vi "Begin.vi"(11 "Image Size":T1=enum."160x120") -> (0 "error out":errorcluster)   [LabVIEW 2012]
doc: "Called before other user functions, this VI is expected to open initial I/O refnums, load in file data, and do all program initialization. Notice that the <B>error out</B> terminal is simply used for data flow. Wiring it to other structures or subVIs ensures that this VI runs first."
uses:
  <vilib>/Rock Robotics/WPI/Camera/WPI_CameraImageSize.ctl
  <vilib>/Rock Robotics/SystemInterfaces/DIO/FPGA_DIOPWMChannel.ctl
  <vilib>/Rock Robotics/WPI/Joystick/WPI_JoystickDeviceEnum.ctl
  <vilib>/Rock Robotics/WPI/Camera/WPI_CameraWhite Balance Values.ctl
  <vilib>/Rock Robotics/WPI/Camera/WPI_CameraExposure Values.ctl
  <vilib>/Rock Robotics/WPI/Camera/WPI_CameraFrameRate.ctl
  <vilib>/Rock Robotics/SystemInterfaces/DIO/FPGA_DIOChannel.ctl
  <vilib>/Rock Robotics/SystemInterfaces/Typedef/FPGA_TypedefDigitalModule.ctl
  <vilib>/Rock Robotics/WPI/Encoder/WPI_EncoderType.ctl
  <vilib>/Rock Robotics/SystemInterfaces/DIO/FPGA_DIORelayChannel.ctl
  <vilib>/Rock Robotics/SystemInterfaces/Typedef/FPGA_TypedefAnalogModuleForGyro.ctl
  <vilib>/Rock Robotics/SystemInterfaces/AI/FPGA_AIGyroChannel.ctl
  <vilib>/Rock Robotics/WPI/Relay/WPI_RelayDirection.ctl
  <vilib>/Rock Robotics/WPI/MotorControl/WPI_MotorControlOpen Victor.vi
  <vilib>/Rock Robotics/WPI/RobotDrive/WPI_RobotDriveOpen4MotorWithJaguar.vi
  Robot Global Data.vi
  <vilib>/Rock Robotics/WPI/Counter/WPI_CounterOpen UpDown Mode.vi
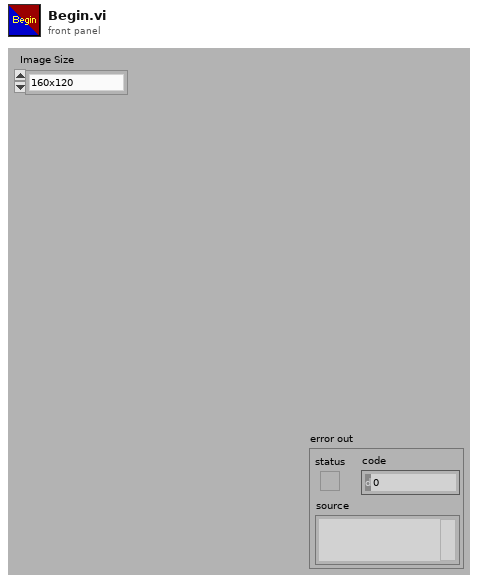
[diagram p1: front panel]
types:
  T1 = typedef "WPI_CameraImageSize.ctl" = enum16{"640x480", "320x240", "160x120"}
  T2 = typedef "FPGA_TypedefDigitalModule.ctl" = enum16{"Digital Module 1", "Digital Module 2"}
  T3 = typedef "FPGA_DIOChannel.ctl" = enum8{"DIO 1", "DIO 2", "DIO 3", "DIO 4", "DIO 5", "DIO 6", "DIO 7", "DIO 8", "DIO 9", "DIO 10", "DIO 11", "DIO 12", "DIO 13", "DIO 14", "Invalid"}
  T4 = typedef "WPI_RelayDirection.ctl" = enum16{"Both directions", "Forward only", "Reverse only"}
  T5 = typedef "FPGA_AIGyroChannel.ctl" = enum8{"AI 1", "AI 2", "Invalid"}
  T6 = typedef "FPGA_TypedefAnalogModuleForGyro.ctl" = enum16{"Analog Module 1"}
  T7 = typedef "FPGA_DIORelayChannel.ctl" = enum8{"Relay 1", "Relay 2", "Relay 3", "Relay 4", "Relay 5", "Relay 6", "Relay 7", "Relay 8", "Invalid"}
  T8 = typedef "WPI_EncoderType.ctl" = enum16{"1x", "2x", "4x"}
  T9 = typedef "FPGA_DIOPWMChannel.ctl" = enum8{"PWM 1", "PWM 2", "PWM 3", "PWM 4", "PWM 5", "PWM 6", "PWM 7", "PWM 8", "PWM 9", "PWM 10", "Invalid"}
  T10 = typedef "WPI_JoystickDeviceEnum.ctl" = enum16{"USB 1", "USB 2", "USB 3", "USB 4", "Kinect 1", "Kinect 2"}
  T11 = typedef "WPI_CameraFrameRate.ctl" = u32
  T12 = typedef "WPI_CameraExposure Values.ctl" = enum16{"Auto", "Flicker-free 50 Hz", "Flicker-free 60 Hz", "Hold current"}
  T13 = typedef "WPI_CameraWhite Balance Values.ctl" = enum16{"Auto", "Fixed indoor", "Fixed outdoor 1", "Fixed outdoor 2", "Fixed fluorescent 1", "Fixed fluorescent 2", "Hold current"}
  T14 = typedef "WPI_CameraDevRef.ctl" = cluster{"Camera Address":string, "CameraStatus":errorcluster, "Acquire Image Notifier":refnum<notifier>}
  T15 = typedef "WPI_DigitalInputDevRef.ctl" = cluster{"DevStatus":errorcluster, "DIO Channel":T3, "Digital Module":T2}
  T16 = typedef "WPI_RobotDriveDevRef.ctl" = cluster{"DevStatus":errorcluster, "Motors[]":T17[], "Square Inputs":bool, "Max Output":dbl, "Isochronous":bool}
  T17 = typedef "WPI_MotorControlDeviceRef.ctl" = cluster{"DeviceStatus":errorcluster, "Type":enum16{"PWM", "CAN"}, "PWM":cluster{"Digital Module":T2, "PWM Channel":T9, "DeadBand":T18}, "CAN":cluster{"Device Number":u8, "Control Mode":T19, "Semaphore":T20, "Max Vout":dbl}, "Invert":bool, "TransformRef":T21, "InvTransformRef":T21}
  T18 = typedef "WPI_PWMDeadband.ctl" = cluster{"Name":string, "maxPositivePwm":i32, "minPositivePwm":i32, "centerPwm":i32, "maxNegativePwm":i32, "minNegativePwm":i32, "angularRange":u16}
  T19 = typedef "WPI_CANJaguar_ControlMode.ctl" = enum8{"Percent VBus", "Current", "Speed", "Position", "Voltage"}
  T20 = typedef "Semaphore RefNum" = refnum<k1>
  T21 = typedef "WPI_PWMTransform_ConPane.ctl" = refnum<vi>
  T22 = typedef "FPGA_CounterEncoderSourceConvertionLVSourceType.ctl" = cluster{"DevStatus":errorcluster, "AnalogTriggerMode?":bool, "DigitalMode":cluster{"Digital Module":T2, "DIO Channel":T23}, "AnalogTriggerMode":cluster{"AnalogTriggerIndex":T24, "OutputType":T25}}
  T23 = typedef "FPGA_DIODigitalSourceChannel.ctl" = enum8{"DIO 1", "DIO 2", "DIO 3", "DIO 4", "DIO 5", "DIO 6", "DIO 7", "DIO 8", "DIO 9", "DIO 10", "DIO 11", "DIO 12", "DIO 13", "DIO 14", "Disabled"}
  T24 = typedef "FPGA_AnalogTriggerIndex.ctl" = enum8{"Trig 0", "Trig 1", "Trig 2", "Trig 3", "Trig 4", "Trig 5", "Trig 6", "Trig 7", "Invalid"}
  T25 = typedef "FPGA_AnalogTriggerOutType.ctl" = enum16{"InWindow", "TriggerState", "Rising", "Falling"}
  T26 = typedef "WPI_GyroDevRef.ctl" = cluster{"DevStatus":errorcluster, "Analog Module":T27, "Analog Channel":T28, "Offset":dbl, "Gain (VoltsPerDegree/Second)":dbl}
  T27 = typedef "FPGA_TypedefAnalogModule.ctl" = enum16{"Analog Module 1", "Analog Module 2"}
  T28 = typedef "FPGA_AIChannel.ctl" = enum8{"AI 1", "AI 2", "AI 3", "AI 4", "AI 5", "AI 6", "AI 7", "AI 8", "Invalid"}
  T29 = typedef "WPI_CounterDevRef.ctl" = cluster{"DevStatus":errorcluster, "CntIndex":T30}
  T30 = typedef "FPGA_CounterCtrSystemIndex.ctl" = enum8{"Ctr 0", "Ctr 1", "Ctr 2", "Ctr 3", "Ctr 4", "Ctr 5", "Ctr 6", "Ctr 7", "Invalid"}
  T31 = typedef "WPI_EncoderDevRef.ctl" = cluster{"DevStatus":errorcluster, "EncoderIndex":T32, "CounterIndex":T30, "DistancePerCount":dbl, "Decoding Type":T8}
  T32 = typedef "FPGA_EncoderIdx.ctl" = enum8{"Enc 0", "Enc 1", "Enc 2", "Enc 3", "Invalid"}
  T33 = typedef "WPI_RelayDevRef.ctl" = cluster{"DevStatus":errorcluster, "Relay Channel":T7, "Digital Module":T2, "Relay Direction":T4}
  T34 = typedef "WPI_JoystickDevRef.ctl" = cluster{"Device":T10}
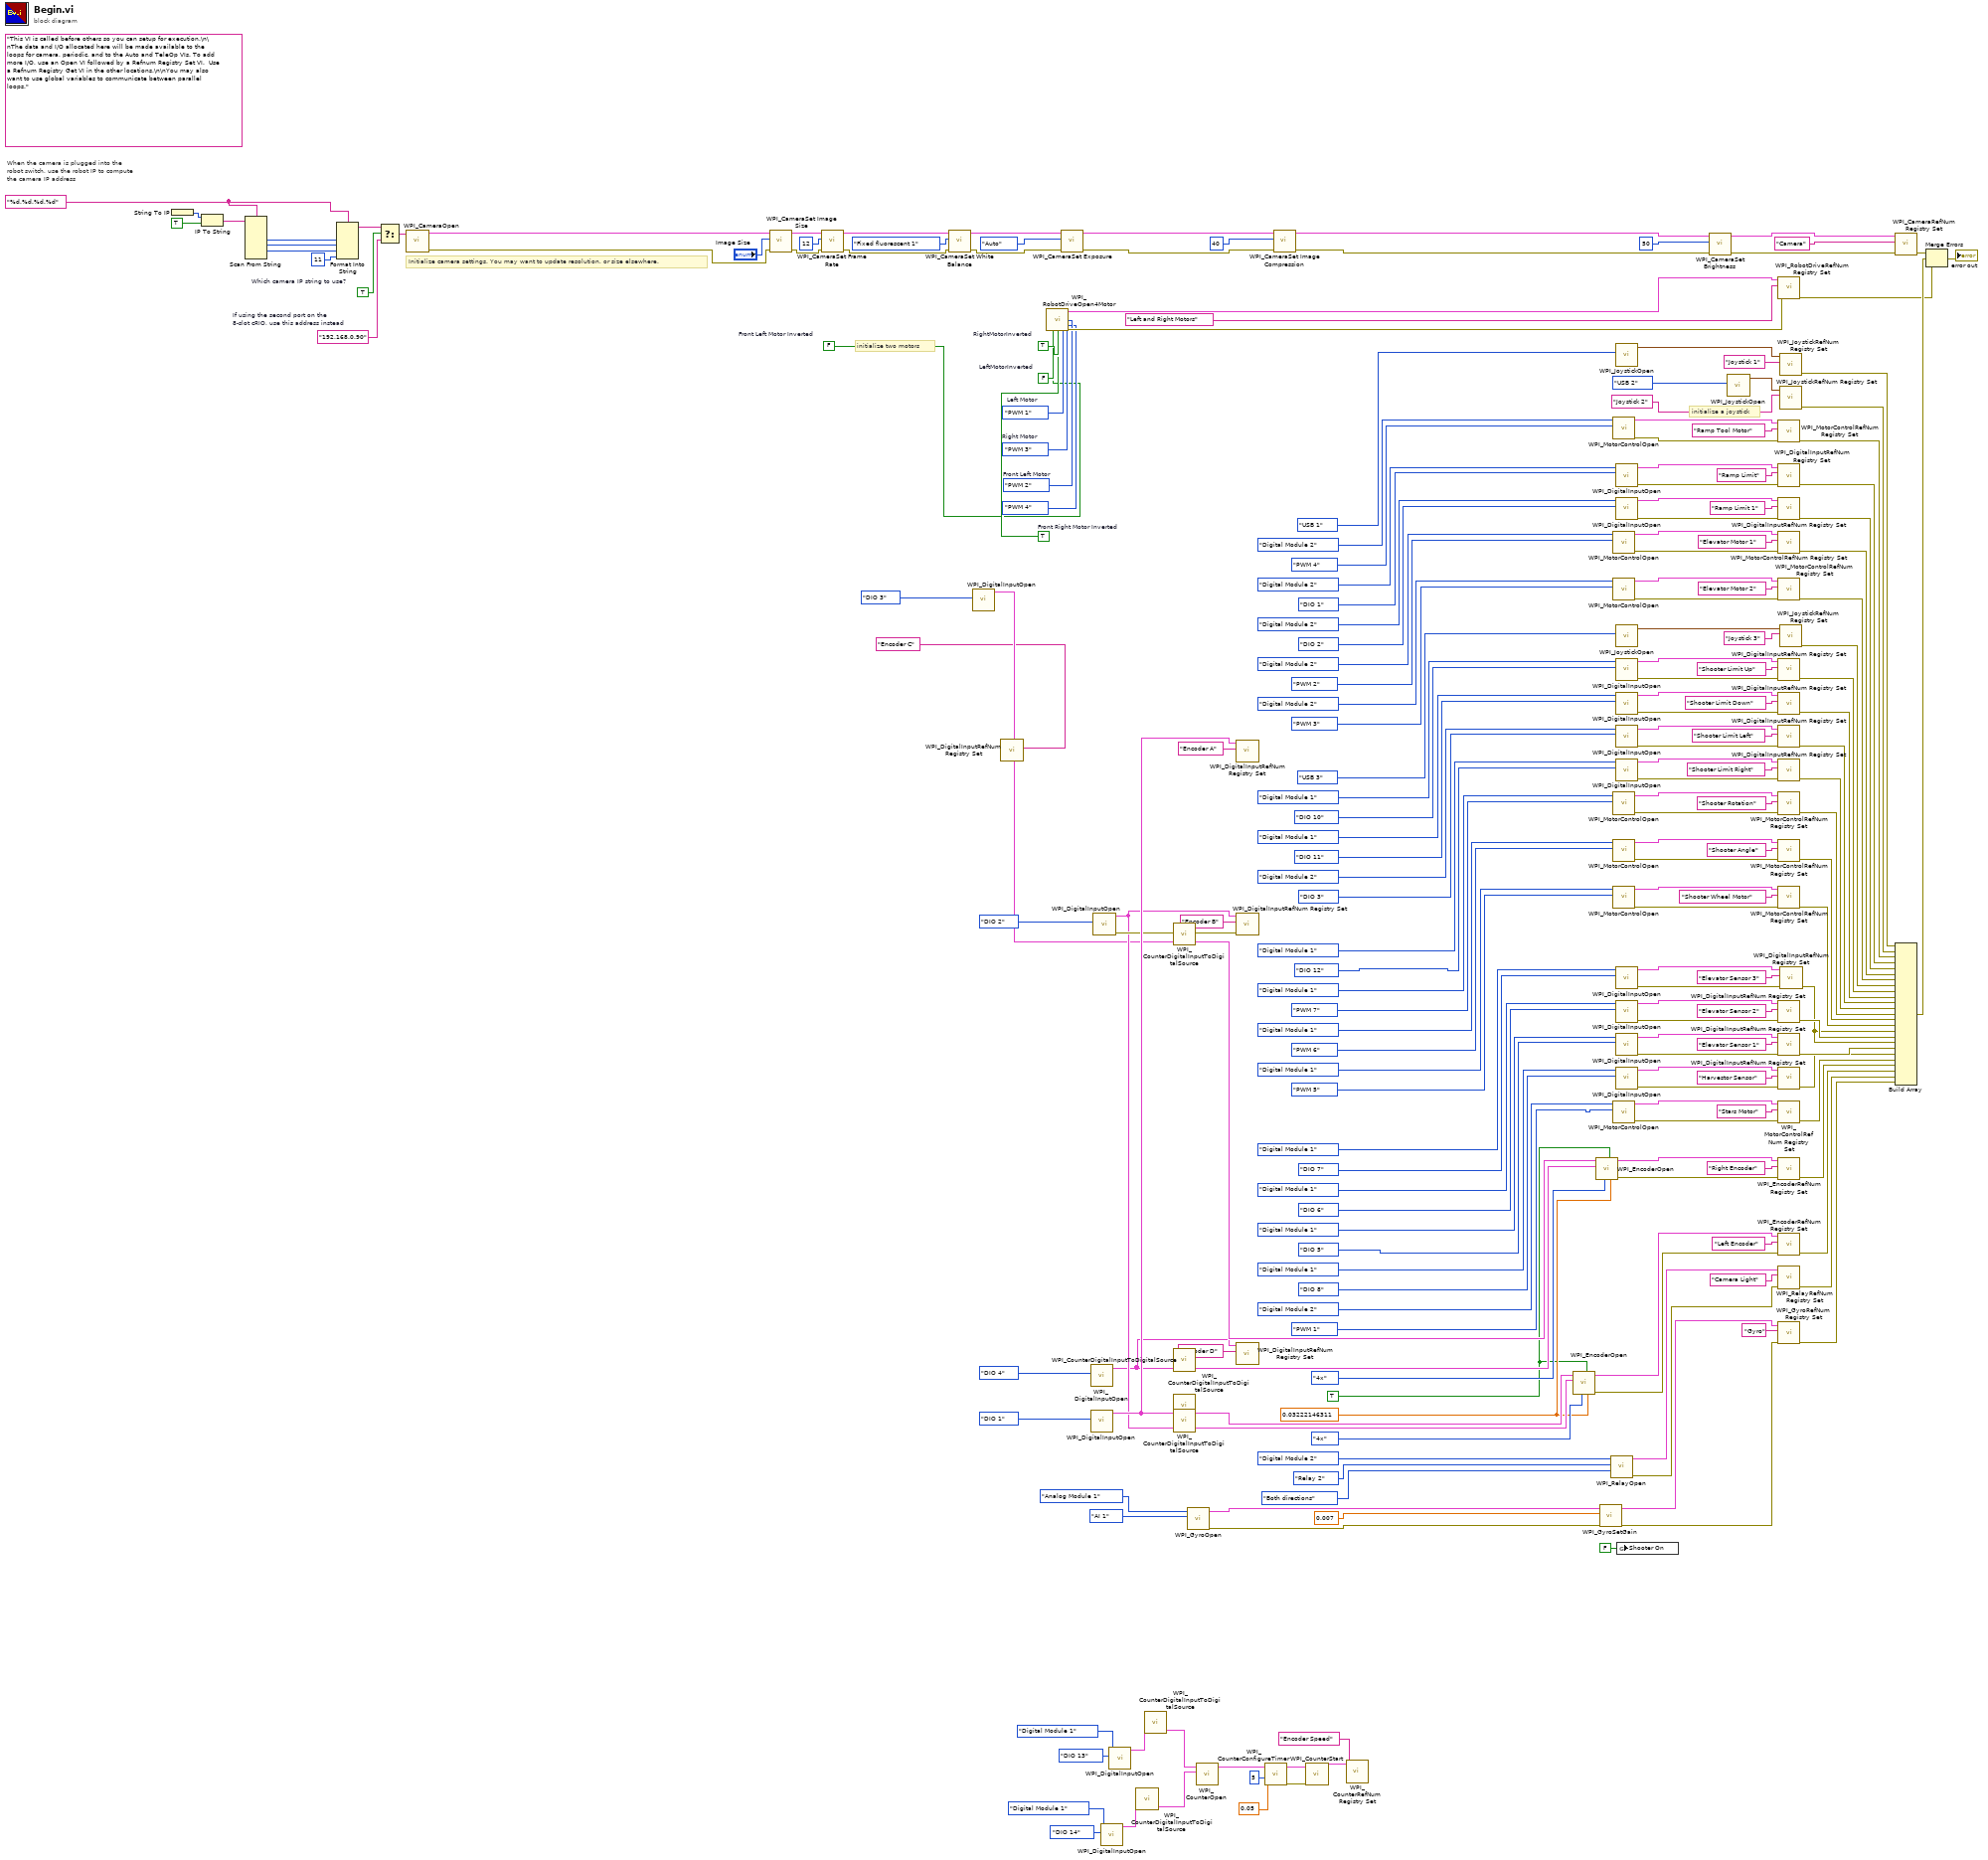
[diagram p0: block diagram]
diagram:
  w25 = FALSE  # Front Left Motor Inverted
  w26 = TRUE  # Front Right Motor Inverted
  w67 = TRUE ("External Reset Active High")
  w77 = 0.03222146311 ("DistancePerCount")
  w163 = FPGA_DIOPWMChannel."PWM 2"  # Front Left Motor
  w181 = TRUE  # Which camera IP string to use?
  w185 = "%d.%d.%d.%d" ("format string")
  (unwired) "This VI is called before others so you can setup for execution.\n\nThe data and I/O allocated here will be made available to the loops for camera, periodic, and to the Auto and TeleOp VIs. To add more I/O, use an Open VI followed by a Refnum Registry Set VI.  Use a Refnum Registry Get VI in the other locations.\n\nYou may also want to use global variables to communicate between parallel loops."
  w197 = FPGA_DIOPWMChannel."PWM 3"  # Right Motor
  w198 = FPGA_DIOPWMChannel."PWM 1"  # Left Motor
  w182 = "192.168.0.90"  # If using the second port on the 8-slot cRIO, use this address instead
  w222 = FALSE  # LeftMotorInverted
  w223 = TRUE  # RightMotorInverted
  # "When the camera is plugged into the\nrobot switch, use the robot IP to compute\nthe camera IP address"
  # "initialize a joystick"
  # "initialize two motors"
  # "Initialize camera settings. You may want to update resolution, or size elsewhere."
  n1 = String To IP() -> (0:w192:u32)  [unwired: 1 in]
  n2 = IP To String(1:TRUE ("dot notation? (F)"), 2:w192) -> (0:w190:string)
  n3 = Scan From String(format string=w185, input string=w190) -> (output 1=w189:i32, output 2=w188:i32, output 3=w187:i32)  [unwired: 7 in, 3 out]
  n4 = Format Into String(format string=w185, w189, w188, w187, 11 ("Compression")) -> (resulting string=w183:string)  [unwired: 2 in, 1 out]
  n5 = Select(t=w183, s=w181, f=w182) -> (s? t:f=w184:string)
  n6 = call <vilib>:"WPI_CameraOpen.vi"("Camera Address"=w184) -> ("error out"=w207:errorcluster, "CameraDevRef"=w208:T14)  [unwired: 2 in, 7 out]
  n7 = call <vilib>:"WPI_CameraSet Image Size.vi"("error in (no error)"=w207, "Image Size"="Image Size", "CameraDevRef"=w208) -> ("error out"=w206:errorcluster, "CameraDevRef Out"=w209:T14)  [unwired: 7 out]
  n8 = call <vilib>:"WPI_CameraSet Frame Rate.vi"("error in (no error)"=w206, "Frame Rate (fps)"=T11 12, "CameraDevRef"=w209) -> ("error out"=w205:errorcluster, "CameraDevRef Out"=w211:T14)  [unwired: 7 out]
  n9 = call <vilib>:"WPI_CameraSet White Balance.vi"("error in (no error)"=w205, "White Balance"=WPI_CameraWhite_Balance_Values."Fixed fluorescent 1", "CameraDevRef"=w211) -> ("error out"=w204:errorcluster, "CameraDevRef Out"=w210:T14)  [unwired: 7 out]
  n10 = call <vilib>:"WPI_DigitalInputOpen.vi"("DIO Channel"=FPGA_DIOChannel."DIO 3") -> ("DigitalInputDevRef"=w71:T15)  [unwired: 2 in, 8 out]
  n11 = call <vilib>:"WPI_DigitalInputRefNum Registry Set.vi"("refnum name"="Encoder C", "DigitalInputDevRef"=w71) -> ()  [unwired: 1 in, 9 out]
  n12 = call-poly <vilib>:"WPI_RobotDriveOpen4Motor.vi"("Rear Left Motor"=w198, "Rear Left Motor Inverted"=w222, "Rear Right Motor Inverted"=w223, "Rear Right Motor"=w197, "Front Left Motor"=w163, "Front Right Motor"=FPGA_DIOPWMChannel."PWM 4", "Front Left Motor Inverted"=w25, "Front Right Motor Inverted"=w26) -> ("RobotDriveDevRef"=w220:T16, "error out"=w216:errorcluster)  [unwired: 6 in]
  n13 = call <vilib>:"WPI_CameraSet Exposure.vi"("error in (no error)"=w204, "Exposure"=WPI_CameraExposure_Values."Auto", "CameraDevRef"=w210) -> ("error out"=w203:errorcluster, "CameraDevRef Out"=w213:T14)  [unwired: 7 out]
  n14 = call <vilib>:"WPI_DigitalInputOpen.vi"("DIO Channel"=FPGA_DIOChannel."DIO 4") -> ("DigitalInputDevRef"=w70:T15)  [unwired: 2 in, 8 out]
  n15 = call <vilib>:"WPI_DigitalInputOpen.vi"("DIO Channel"=FPGA_DIOChannel."DIO 1") -> ("DigitalInputDevRef"=w76:T15)  [unwired: 2 in, 8 out]
  n16 = call <vilib>:"WPI_DigitalInputOpen.vi"("DIO Channel"=FPGA_DIOChannel."DIO 2") -> ("error out"=w74:errorcluster, "DigitalInputDevRef"=w73:T15)  [unwired: 2 in, 7 out]
  n17 = call <vilib>:"WPI_DigitalInputOpen.vi"("DIO Channel"=FPGA_DIOChannel."DIO 14", "Digital Module (Module 1)"=FPGA_TypedefDigitalModule."Digital Module 1") -> ("DigitalInputDevRef"=w9:T15)  [unwired: 8 in, 1 out]
  n18 = call <vilib>:"WPI_DigitalInputOpen.vi"("DIO Channel"=FPGA_DIOChannel."DIO 13", "Digital Module (Module 1)"=FPGA_TypedefDigitalModule."Digital Module 1") -> ("DigitalInputDevRef"=w13:T15)  [unwired: 8 in, 1 out]
  n19 = call <vilib>:"WPI_CounterDigitalInputToDigitalSource.vi"("DigitalInputDevRef"=w9) -> ("Digital Source"=w8:T22)  [unwired: 6 out]
  n20 = call <vilib>:"WPI_CounterDigitalInputToDigitalSource.vi"("DigitalInputDevRef"=w13) -> ("Digital Source"=w12:T22)  [unwired: 6 out]
  n21 = call <vilib>:"WPI_CounterDigitalInputToDigitalSource.vi"("DigitalInputDevRef"=w71) -> ("Digital Source"=w80:T22)  [unwired: 6 out]
  n22 = call <vilib>:"WPI_CounterDigitalInputToDigitalSource.vi"("DigitalInputDevRef"=w70) -> ("Digital Source"=w78:T22)  [unwired: 6 out]
  n23 = call <vilib>:"WPI_CounterDigitalInputToDigitalSource.vi"("DigitalInputDevRef"=w76) -> ("Digital Source"=w84:T22)  [unwired: 6 out]
  n24 = call <vilib>:"WPI_CounterDigitalInputToDigitalSource.vi"("DigitalInputDevRef"=w73) -> ("Digital Source"=w83:T22)  [unwired: 6 out]
  n25 = call <vilib>:"WPI_GyroOpen.vi"("Analog Channel"=FPGA_AIGyroChannel."AI 1", "Analog Module (Module 1)"=FPGA_TypedefAnalogModuleForGyro."Analog Module 1" ("Analog Module (Slot 1)")) -> ("error out"=w31:errorcluster, "GyroDevRef"=w35:T26)  [unwired: 4 in, 4 out]
  n26 = call-poly <vilib>:"WPI_CounterOpen.vi"("Down Source"=w8, "Up Source"=w12) -> ("CounterDevRef"=w1:T29)  [unwired: 8 in, 1 out]
  n27 = call <vilib>:"WPI_DigitalInputRefNum Registry Set.vi"("refnum name"="Encoder A", "DigitalInputDevRef"=w76) -> ()  [unwired: 1 in, 9 out]
  n28 = call <vilib>:"WPI_DigitalInputRefNum Registry Set.vi"("error in (no error)"=w74, "refnum name"="Encoder B", "DigitalInputDevRef"=w73) -> ()  [unwired: 9 out]
  n29 = call <vilib>:"WPI_DigitalInputRefNum Registry Set.vi"("refnum name"="Encoder D", "DigitalInputDevRef"=w70) -> ()  [unwired: 1 in, 9 out]
  n30 = call <vilib>:"WPI_CounterConfigureTimer.vi"("Number Samples to Average"=u8 5, "MaxPeriod (sec)"=0.05, "CounterDevRef in"=w1) -> ("error out"=w7:errorcluster, "CounterDevRef out"=w6:T29)  [unwired: 7 in]
  n31 = call <vilib>:"WPI_CameraSet Image Compression.vi"("error in (no error)"=w203, "Compression"=40, "CameraDevRef"=w213) -> ("error out"=w202:errorcluster, "CameraDevRef Out"=w212:T14)  [unwired: 7 out]
  n32 = call <vilib>:"WPI_CounterStart.vi"("error in (no error)"=w7, "CounterDevRef in"=w6) -> ("CounterDevRef out"=w5:T29)  [unwired: 8 in, 1 out]
  n33 = call <vilib>:"WPI_CounterRefNum Registry Set.vi"("refnum name"="Encoder Speed", "CounterDevRef"=w5) -> ()  [unwired: 8 in, 2 out]
  n34 = call <vilib>:"WPI_EncoderOpen.vi"("DistancePerCount"=w77, "External Reset Active High"=w67, "Decoding Type"=WPI_EncoderType."4x", "BSource"=w83, "ASource"=w84) -> ("error out"=w92:errorcluster, "EncoderDevRef"=w91:T31)  [unwired: 3 in, 2 out]
  n35 = call <vilib>:"WPI_EncoderOpen.vi"("DistancePerCount"=w77, "External Reset Active High"=w67, "Decoding Type"=WPI_EncoderType."4x", "BSource"=w78, "ASource"=w80) -> ("error out"=w90:errorcluster, "EncoderDevRef"=w89:T31)  [unwired: 3 in, 2 out]
  n36 = call <vilib>:"WPI_GyroSetGain.vi"("error in (no error)"=w31, "Gain (VoltsPerDegree/Second)"=0.007, "GyroDevRef"=w35) -> ("error out"=w30:errorcluster, "GyroDevRef"=w32:T26)  [unwired: 7 out]
  n37 = call <vilib>:"WPI_RelayOpen.vi"("Relay Direction"=WPI_RelayDirection."Both directions", "Relay Channel"=FPGA_DIORelayChannel."Relay 2", "Digital Module (Module 1)"=FPGA_TypedefDigitalModule."Digital Module 2") -> ("error out"=w39:errorcluster, "RelayDevRef"=w40:T33)  [unwired: 7 in]
  n38 = call-poly <vilib>:"WPI_MotorControlOpen.vi"("PWM Channel"=FPGA_DIOPWMChannel."PWM 4", "Digital Module (Module 1)"=FPGA_TypedefDigitalModule."Digital Module 2") -> ("error out"=w176:errorcluster, "MotorControlDeviceRef"=w177:T17)  [unwired: 8 in]
  n39 = call-poly <vilib>:"WPI_MotorControlOpen.vi"("PWM Channel"=FPGA_DIOPWMChannel."PWM 2", "Digital Module (Module 1)"=FPGA_TypedefDigitalModule."Digital Module 2") -> ("error out"=w159:errorcluster, "MotorControlDeviceRef"=w161:T17)  [unwired: 8 in]
  n40 = call-poly <vilib>:"WPI_MotorControlOpen.vi"("PWM Channel"=FPGA_DIOPWMChannel."PWM 3", "Digital Module (Module 1)"=FPGA_TypedefDigitalModule."Digital Module 2") -> ("error out"=w156:errorcluster, "MotorControlDeviceRef"=w158:T17)  [unwired: 8 in]
  n41 = call-poly <vilib>:"WPI_MotorControlOpen.vi"("PWM Channel"=FPGA_DIOPWMChannel."PWM 7", "Digital Module (Module 1)"=FPGA_TypedefDigitalModule."Digital Module 1") -> ("error out"=w132:errorcluster, "MotorControlDeviceRef"=w133:T17)  [unwired: 8 in]
  n42 = call-poly <vilib>:"WPI_MotorControlOpen.vi"("PWM Channel"=FPGA_DIOPWMChannel."PWM 6", "Digital Module (Module 1)"=FPGA_TypedefDigitalModule."Digital Module 1") -> ("error out"=w127:errorcluster, "MotorControlDeviceRef"=w128:T17)  [unwired: 8 in]
  n43 = call-poly <vilib>:"WPI_MotorControlOpen.vi"("PWM Channel"=FPGA_DIOPWMChannel."PWM 5", "Digital Module (Module 1)"=FPGA_TypedefDigitalModule."Digital Module 1") -> ("error out"=w123:errorcluster, "MotorControlDeviceRef"=w124:T17)  [unwired: 8 in]
  n44 = call-poly <vilib>:"WPI_MotorControlOpen.vi"("PWM Channel"=FPGA_DIOPWMChannel."PWM 1", "Digital Module (Module 1)"=FPGA_TypedefDigitalModule."Digital Module 2") -> ("error out"=w95:errorcluster, "MotorControlDeviceRef"=w96:T17)  [unwired: 8 in]
  n45 = call <vilib>:"WPI_JoystickOpen.vi"("JoystickDevice"=WPI_JoystickDeviceEnum."USB 1") -> ("JoystickDevRef"=w218:T34)  [unwired: 10 out]
  n46 = call <vilib>:"WPI_DigitalInputOpen.vi"("DIO Channel"=FPGA_DIOChannel."DIO 1", "Digital Module (Module 1)"=FPGA_TypedefDigitalModule."Digital Module 2") -> ("error out"=w172:errorcluster, "DigitalInputDevRef"=w171:T15)  [unwired: 8 in]
  n47 = call <vilib>:"WPI_DigitalInputOpen.vi"("DIO Channel"=FPGA_DIOChannel."DIO 2", "Digital Module (Module 1)"=FPGA_TypedefDigitalModule."Digital Module 2") -> ("error out"=w168:errorcluster, "DigitalInputDevRef"=w167:T15)  [unwired: 8 in]
  n48 = call <vilib>:"WPI_JoystickOpen.vi"("JoystickDevice"=WPI_JoystickDeviceEnum."USB 3") -> ("JoystickDevRef"=w151:T34)  [unwired: 10 out]
  n49 = call <vilib>:"WPI_DigitalInputOpen.vi"("DIO Channel"=FPGA_DIOChannel."DIO 10", "Digital Module (Module 1)"=FPGA_TypedefDigitalModule."Digital Module 1") -> ("error out"=w115:errorcluster, "DigitalInputDevRef"=w148:T15)  [unwired: 8 in]
  n50 = call <vilib>:"WPI_DigitalInputOpen.vi"("DIO Channel"=FPGA_DIOChannel."DIO 11", "Digital Module (Module 1)"=FPGA_TypedefDigitalModule."Digital Module 1") -> ("error out"=w114:errorcluster, "DigitalInputDevRef"=w144:T15)  [unwired: 8 in]
  n51 = call <vilib>:"WPI_DigitalInputOpen.vi"("DIO Channel"=FPGA_DIOChannel."DIO 3", "Digital Module (Module 1)"=FPGA_TypedefDigitalModule."Digital Module 2") -> ("error out"=w113:errorcluster, "DigitalInputDevRef"=w140:T15)  [unwired: 8 in]
  n52 = call <vilib>:"WPI_DigitalInputOpen.vi"("DIO Channel"=FPGA_DIOChannel."DIO 12", "Digital Module (Module 1)"=FPGA_TypedefDigitalModule."Digital Module 1") -> ("error out"=w112:errorcluster, "DigitalInputDevRef"=w136:T15)  [unwired: 8 in]
  n53 = call <vilib>:"WPI_DigitalInputOpen.vi"("DIO Channel"=FPGA_DIOChannel."DIO 7", "Digital Module (Module 1)"=FPGA_TypedefDigitalModule."Digital Module 1") -> ("error out"=w111:errorcluster, "DigitalInputDevRef"=w119:T15)  [unwired: 8 in]
  n54 = call <vilib>:"WPI_DigitalInputOpen.vi"("DIO Channel"=FPGA_DIOChannel."DIO 6", "Digital Module (Module 1)"=FPGA_TypedefDigitalModule."Digital Module 1") -> ("error out"=w106:errorcluster, "DigitalInputDevRef"=w110:T15)  [unwired: 8 in]
  n55 = call <vilib>:"WPI_DigitalInputOpen.vi"("DIO Channel"=FPGA_DIOChannel."DIO 5", "Digital Module (Module 1)"=FPGA_TypedefDigitalModule."Digital Module 1") -> ("error out"=w102:errorcluster, "DigitalInputDevRef"=w105:T15)  [unwired: 8 in]
  n56 = call <vilib>:"WPI_DigitalInputOpen.vi"("DIO Channel"=FPGA_DIOChannel."DIO 8", "Digital Module (Module 1)"=FPGA_TypedefDigitalModule."Digital Module 1") -> ("error out"=w97:errorcluster, "DigitalInputDevRef"=w101:T15)  [unwired: 8 in]
  n57 = global write "Robot Global Data.vi" "Shooter On"(FALSE ("Shooter On")) -> ()
  n58 = call <vilib>:"WPI_CameraSet Brightness.vi"("error in (no error)"=w202, "Brightness"=50, "CameraDevRef"=w212) -> ("error out"=w200:errorcluster, "CameraDevRef Out"=w201:T14)  [unwired: 7 out]
  n59 = call <vilib>:"WPI_JoystickOpen.vi"("JoystickDevice"=WPI_JoystickDeviceEnum."USB 2") -> ("JoystickDevRef"=w180:T34)  [unwired: 10 in]
  n60 = call <vilib>:"WPI_RobotDriveRefNum Registry Set.vi"("error in (no error)"=w216, "refnum name"="Left and Right Motors", "RobotDriveDevRef"=w220) -> ("error out"=w17:errorcluster)  [unwired: 8 out]
  n61 = call <vilib>:"WPI_MotorControlRefNum Registry Set.vi"("error in (no error)"=w176, "refnum name"="Ramp Tool Motor", "MotorControlDevRef"=w177) -> ("error out"=w63:errorcluster)  [unwired: 7 in, 1 out]
  n62 = call <vilib>:"WPI_DigitalInputRefNum Registry Set.vi"("error in (no error)"=w172, "refnum name"="Ramp Limit", "DigitalInputDevRef"=w171) -> ("error out"=w62:errorcluster)  [unwired: 7 in, 1 out]
  n63 = call <vilib>:"WPI_DigitalInputRefNum Registry Set.vi"("error in (no error)"=w168, "refnum name"="Ramp Limit 1", "DigitalInputDevRef"=w167) -> ("error out"=w61:errorcluster)  [unwired: 7 in, 1 out]
  n64 = call <vilib>:"WPI_MotorControlRefNum Registry Set.vi"("error in (no error)"=w159, "refnum name"="Elevator Motor 1", "MotorControlDevRef"=w161) -> ("error out"=w60:errorcluster)  [unwired: 7 in, 1 out]
  n65 = call <vilib>:"WPI_MotorControlRefNum Registry Set.vi"("error in (no error)"=w156, "refnum name"="Elevator Motor 2", "MotorControlDevRef"=w158) -> ("error out"=w59:errorcluster)  [unwired: 7 in, 1 out]
  n66 = call <vilib>:"WPI_DigitalInputRefNum Registry Set.vi"("error in (no error)"=w115, "refnum name"="Shooter Limit Up", "DigitalInputDevRef"=w148) -> ("error out"=w57:errorcluster)  [unwired: 7 in, 1 out]
  n67 = call <vilib>:"WPI_DigitalInputRefNum Registry Set.vi"("error in (no error)"=w114, "refnum name"="Shooter Limit Down", "DigitalInputDevRef"=w144) -> ("error out"=w56:errorcluster)  [unwired: 7 in, 1 out]
  n68 = call <vilib>:"WPI_DigitalInputRefNum Registry Set.vi"("error in (no error)"=w113, "refnum name"="Shooter Limit Left", "DigitalInputDevRef"=w140) -> ("error out"=w55:errorcluster)  [unwired: 7 in, 1 out]
  n69 = call <vilib>:"WPI_DigitalInputRefNum Registry Set.vi"("error in (no error)"=w112, "refnum name"="Shooter Limit Right", "DigitalInputDevRef"=w136) -> ("error out"=w54:errorcluster)  [unwired: 7 in, 1 out]
  n70 = call <vilib>:"WPI_MotorControlRefNum Registry Set.vi"("error in (no error)"=w132, "refnum name"="Shooter Rotation", "MotorControlDevRef"=w133) -> ("error out"=w53:errorcluster)  [unwired: 7 in, 1 out]
  n71 = call <vilib>:"WPI_MotorControlRefNum Registry Set.vi"("error in (no error)"=w127, "refnum name"="Shooter Angle", "MotorControlDevRef"=w128) -> ("error out"=w52:errorcluster)  [unwired: 7 in, 1 out]
  n72 = call <vilib>:"WPI_MotorControlRefNum Registry Set.vi"("error in (no error)"=w123, "refnum name"="Shooter Wheel Motor", "MotorControlDevRef"=w124) -> ("error out"=w51:errorcluster)  [unwired: 7 in, 1 out]
  n73 = call <vilib>:"WPI_DigitalInputRefNum Registry Set.vi"("error in (no error)"=w106, "refnum name"="Elevator Sensor 2", "DigitalInputDevRef"=w110) -> ("error out"=w50:errorcluster)  [unwired: 7 in, 1 out]
  n74 = call <vilib>:"WPI_DigitalInputRefNum Registry Set.vi"("error in (no error)"=w102, "refnum name"="Elevator Sensor 1", "DigitalInputDevRef"=w105) -> ("error out"=w48:errorcluster)  [unwired: 7 in, 1 out]
  n75 = call <vilib>:"WPI_DigitalInputRefNum Registry Set.vi"("error in (no error)"=w97, "refnum name"="Harvestor Sensor", "DigitalInputDevRef"=w101) -> ("error out"=w47:errorcluster)  [unwired: 7 in, 1 out]
  n76 = call <vilib>:"WPI_MotorControlRefNum Registry Set.vi"("error in (no error)"=w95, "refnum name"="Stars Motor", "MotorControlDevRef"=w96) -> ("error out"=w46:errorcluster)  [unwired: 7 in, 1 out]
  n77 = call <vilib>:"WPI_EncoderRefNum Registry Set.vi"("error in (no error)"=w90, "refnum name"="Right Encoder", "EncoderDevRef"=w89) -> ("error out"=w45:errorcluster)  [unwired: 8 out]
  n78 = call <vilib>:"WPI_EncoderRefNum Registry Set.vi"("error in (no error)"=w92, "refnum name"="Left Encoder", "EncoderDevRef"=w91) -> ("error out"=w44:errorcluster)  [unwired: 8 out]
  n79 = call <vilib>:"WPI_RelayRefNum Registry Set.vi"("error in (no error)"=w39, "refnum name"="Camera Light", "RelayDevRef"=w40) -> ("error out"=w36:errorcluster)  [unwired: 7 in, 1 out]
  n80 = call <vilib>:"WPI_GyroRefNum Registry Set.vi"("error in (no error)"=w30, "refnum name"="Gyro", "GyroDevRef"=w32) -> ("error out"=w27:errorcluster)  [unwired: 8 out]
  n81 = call <vilib>:"WPI_JoystickRefNum Registry Set.vi"("refnum name"="Joystick 1", "JoystickDevRef"=w218) -> ("error out"=w65:errorcluster)  [unwired: 1 in, 8 out]
  n82 = call <vilib>:"WPI_JoystickRefNum Registry Set.vi"("refnum name"="Joystick 2", "JoystickDevRef"=w180) -> ("error out"=w64:errorcluster)  [unwired: 8 in, 1 out]
  n83 = call <vilib>:"WPI_JoystickRefNum Registry Set.vi"("refnum name"="Joystick 3", "JoystickDevRef"=w151) -> ("error out"=w58:errorcluster)  [unwired: 1 in, 8 out]
  n84 = call <vilib>:"WPI_DigitalInputRefNum Registry Set.vi"("error in (no error)"=w111, "refnum name"="Elevator Sensor 3", "DigitalInputDevRef"=w119) -> ("error out"=w49:errorcluster)  [unwired: 7 in, 1 out]
  n85 = call <vilib>:"WPI_CameraRefNum Registry Set.vi"("error in (no error)"=w200, "refnum name"="Camera", "CameraDevRef"=w201) -> ("error out"=w41:errorcluster)  [unwired: 8 out]
  n86 = Build Array(w65, w64, w63, w62, w61, w60, w59, w58, w57, w56, w55, w54, w53, w52, w51, w49, w50, w49, w48, w47, w46, w45, w44, w36, w27) -> (w42:errorcluster[])
  n87 = Merge Errors(w41, w42, w17) -> (→"error out":errorcluster)
